vi "Compute.vi"(8 "error in (no error)":errorcluster, 9 "Data Channels":T3, 10 "x-var":T2(array[cluster]), 11 "Difference in":refnum<class "Difference.lvclass">) -> (0 "error out":errorcluster, 1 "Add'l Data Channels":T3, 3 "Difference out":refnum<class "Difference.lvclass">)   [LabVIEW 2023, in "Difference.lvclass"]
doc: "Given a data channel and an x-coordinate, compute and return one or more new data channels."
uses:
  Difference.lvclass
  Instruments/Utility Classes/Readable/Data Channels.ctl
  Instruments/Utility Classes/Readable/Data Channel.ctl
  Instruments/Utility Classes/Readable/Data Point.ctl
  Instruments/Utility Classes/Readable/Time.ctl
  Instruments/Utility Classes/Readable/X.ctl
  Instruments/Utility Classes/Readable/Readable.lvclass
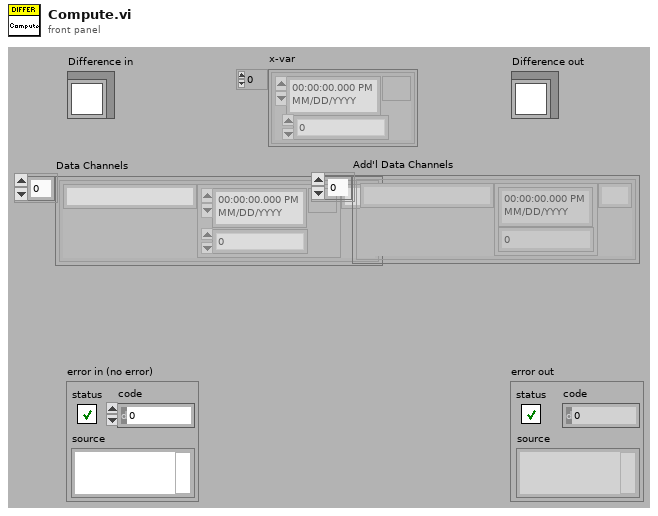
[diagram p1: front panel]
types:
  T1 = typedef "Readable.lvclass/X.ctl" = dbl
  T2 = cluster{"seconds since 1Jan1904":timestamp, "X-Var":T1}[]
  T3 = typedef "Readable.lvclass/Data Channels.ctl" = T4[]
  T4 = typedef "Readable.lvclass/Data Channel.ctl" = cluster{"Name":string, "Data Point":T5, "Unit":string}
  T5 = typedef "Readable.lvclass/Data Point.ctl" = cluster{"t":T6, "x":T1}
  T6 = typedef "Readable.lvclass/Time.ctl" = timestamp
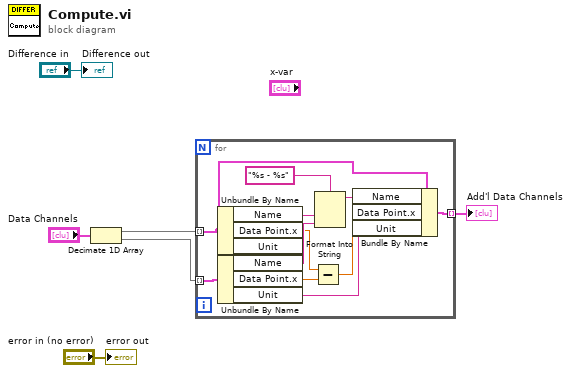
[diagram p0: block diagram]
diagram:
  n1 = Decimate 1D Array "Decimate 1D Array"("Data Channels") -> (w6:T4[], w5:T4[])
  n2 = for {
    tunnel: w6 -> [w13] mode=indexing
    tunnel: w5 -> [w17] mode=indexing
    tunnel: [w7] -> w3 mode=indexing
    n3 = Unbundle By Name(w13) -> ("Name"=w15:string, "Data Point.x"=w10:T1)  [unwired: 1 out]
    n4 = Unbundle By Name(w17) -> ("Name"=w14:string, "Data Point.x"=w9:T1, "Unit"=w12:string)
    n5 = Subtract(x=w10, y=w9) -> (x-y=w8:T1)
    n6 = Format Into String(format string="%s - %s", w15, w14) -> (resulting string=w11:string)  [unwired: 2 in, 1 out]
    n7 = Bundle By Name(cluster=w13, "Name"=w11, "Data Point.x"=w8, "Unit"=w12) -> (w7:T4)
  }
  "Add'l Data Channels" <- w3
  "error out" <- "error in (no error)"
  "Difference out" <- "Difference in"
